vi "Script Add Custom Error.vi"(5 "Error Code":i32, 6 "Error Description":string, 7 "Error Name":string="TESTING.vi", 8 "error in":errorcluster, 9 "Error Arguments Window Ref":refnum<vi>, 10 "DQMH Lib Ref":refnum<vi>, 11 "Module type":T1) -> (0 "error out":errorcluster)   [LabVIEW 2019, in "Panther Dashboard.lvlib"]
uses:
  Panther Dashboard.lvlib
  Module type--enum.ctl
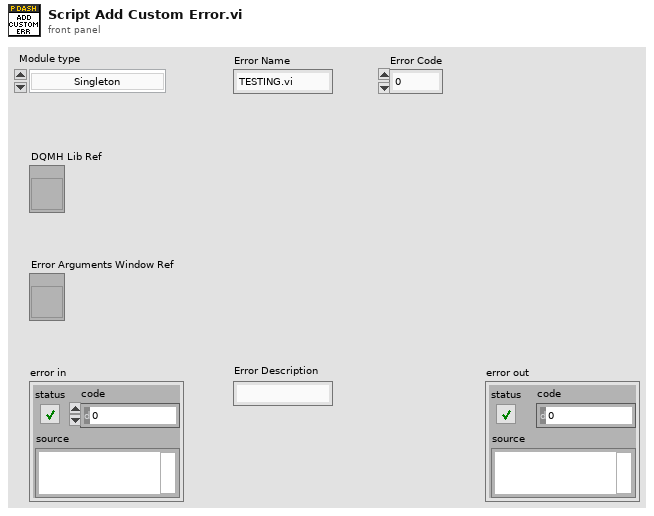
[diagram p1: front panel]
types:
  T1 = typedef "Panther Dashboard.lvlib/Module type--enum.ctl" = enum16{"Singleton", "Cloneable"}
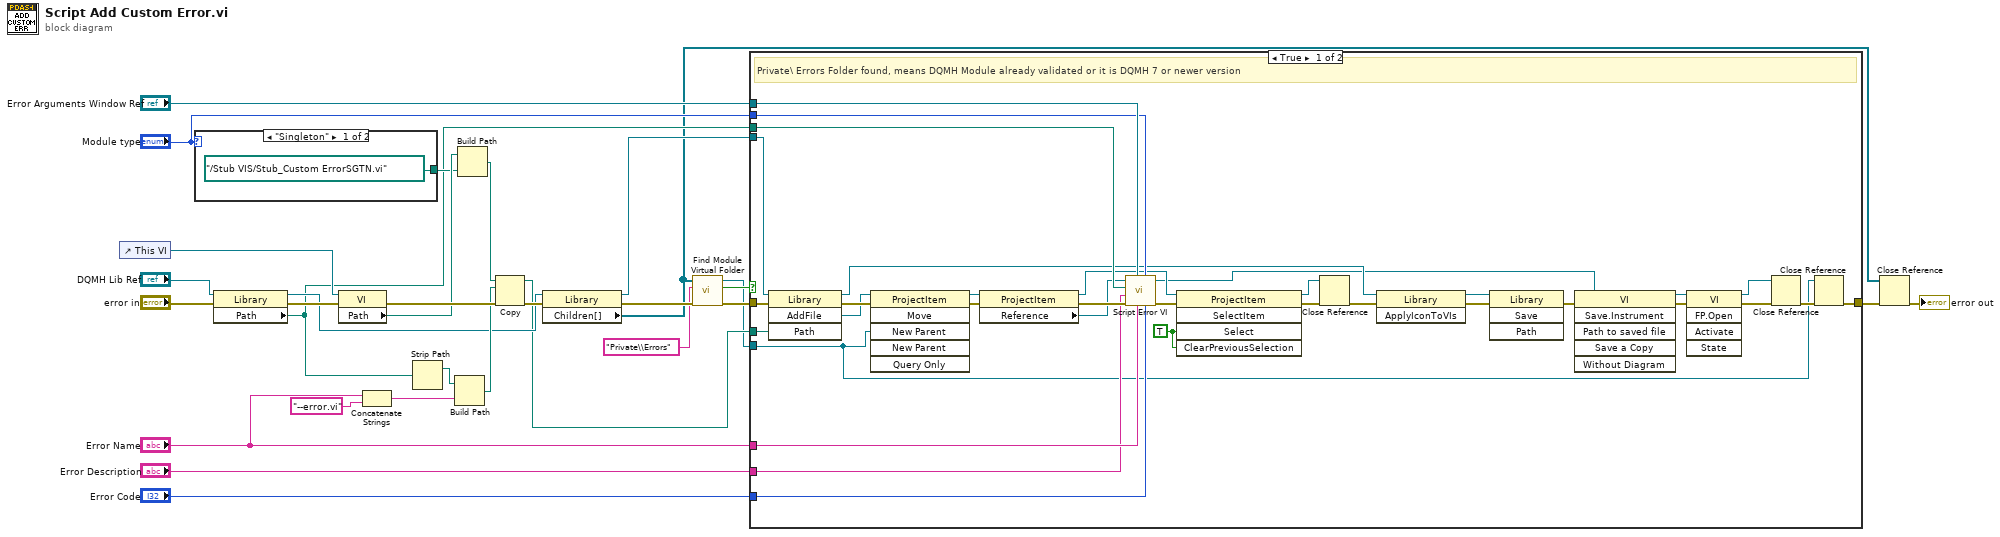
[diagram p0: block diagram]
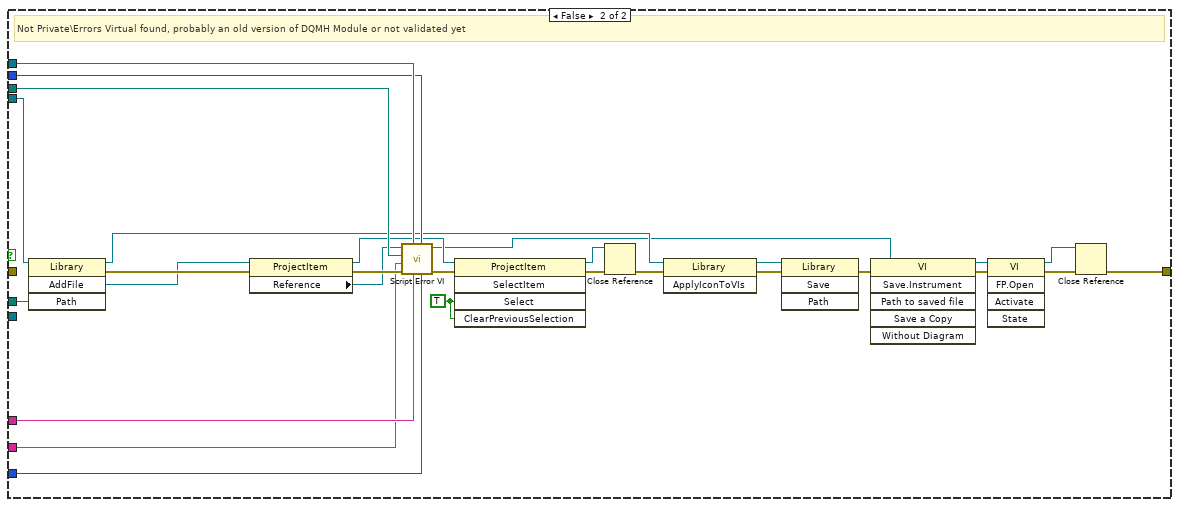
[diagram p2: hidden frame]
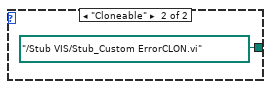
[diagram p3: hidden frame]
diagram:
  n1 = control-ref of="This VI"() -> (w20:refnum<vi>)
  n2 = case shown="\"Singleton\"" "Module type" {
    tunnel: [path "../Stub VIS/Stub_Custom ErrorSGTN.vi" path "../Stub VIS/Stub_Custom ErrorCLON.vi"] -> w18
    frame "Singleton" {
    }
    frame "Cloneable" {
    }
  }
  n3 = property class="Library"(reference="DQMH Lib Ref", error in="error in") -> (reference out=w13:refnum<vi>, error out=w28:errorcluster, "Path"=w11:path)
  n4 = property class="VI"(reference=w20, error in=w28) -> (error out=w29:errorcluster, "Path"=w19:path)  [unwired: 1 out]
  n5 = Concatenate Strings("Error Name", "--error.vi" ("input 1")) -> (w22:string)
  n6 = Strip Path(path=w11) -> (stripped path=w14:path)  [unwired: 1 out]
  n7 = Build Path(base path=w14, name or relative path=w22) -> (appended path=w21:path)
  n8 = Build Path(base path=w19, name or relative path=w18) -> (appended path=w17:path)
  n9 = Copy(8:w29, 10:w21, 11:w17) -> (0:w27:errorcluster, 3:w12:path)  [unwired: 2 in, 1 out]
  n10 = property class="Library"(reference=w13, error in=w27) -> (reference out=w16:refnum<vi>, error out=w24:errorcluster, "Children[]"=w4:refnum<vi>[])
  n11 = call "Find Module Virtual Folder.vi"("error in"=w24, "Virtual Folder"="Private\\Errors", "Children[]"=w4) -> ("error out"=w23:errorcluster, "Found?"=w3:bool, "ProjectItem out"=w2:refnum<vi>)  [unwired: 6 in]
  n12 = case shown="True" w3 {
    tunnel: [w63 w85] -> w30
    tunnel: w16 -> [w51 w82]
    tunnel: w12 -> [w52 w83]
    tunnel: w11 -> [w48 w80]
    tunnel: "Error Name" -> [w40 w72]
    tunnel: "Error Code" -> [w47 w79]
    tunnel: "Error Arguments Window Ref" -> [w45 w77]
    tunnel: "Module type" -> [w44 w76]
    tunnel: "Error Description" -> [w34 w66]
    tunnel: w2 -> [w33 _]
    tunnel: w23 -> [w53 _]
    frame True {
      w41 = TRUE ("Select")
      # "Private\\ Errors Folder found, means DQMH Module already validated or it is DQMH 7 or newer version"
      n13 = invoke class="Library" method="AddFile"(reference=w51, error in=w53, "Path"=w52) -> (reference out=w39:refnum<vi>, error out=w64:errorcluster, "AddFile"=w50:refnum<vi>)  [unwired: 1 in, 1 out]
      n14 = invoke class="ProjectItem" method="Move"(reference=w50, error in=w64, "New Parent"=w33) -> (reference out=w49:refnum<vi>, error out=w65:errorcluster)  [unwired: 3 in, 4 out]
      n15 = property class="ProjectItem"(reference=w49, error in=w65) -> (reference out=w43:refnum<vi>, error out=w60:errorcluster, "Reference"=w46:refnum<vi>)
      n16 = call "Script Error VI.vi"("Error Code"=w47, "Module type"=w44, "Error Name"=w40, "Error Arguments Window Ref"=w45, "error in"=w60, "Error Description"=w34, "Library Path"=w48, "VI Ref Error in"=w46) -> ("error out"=w62:errorcluster, "Custom Error VI Ref"=w36:refnum<vi>)  [unwired: 2 in]
      n17 = invoke class="ProjectItem" method="SelectItem"(reference=w43, error in=w62, "Select"=w41, "ClearPreviousSelection"=w41) -> (reference out=w42:refnum<vi>, error out=w61:errorcluster)  [unwired: 1 in, 3 out]
      n18 = Close Reference(reference=w42, error in (no error)=w61) -> (error out=w59:errorcluster)
      n19 = invoke class="Library" method="ApplyIconToVIs"(reference=w39, error in=w59) -> (reference out=w38:refnum<vi>, error out=w58:errorcluster)  [unwired: 1 in, 1 out]
      n20 = invoke class="Library" method="Save"(reference=w38, error in=w58) -> (error out=w57:errorcluster)  [unwired: 2 in, 3 out]
      n21 = invoke class="VI" method="Save.Instrument"(reference=w36, error in=w57) -> (reference out=w35:refnum<vi>, error out=w54:errorcluster)  [unwired: 4 in, 4 out]
      n22 = invoke class="VI" method="FP.Open"(reference=w35, error in=w54) -> (reference out=w37:refnum<vi>, error out=w56:errorcluster)  [unwired: 3 in, 3 out]
      n23 = Close Reference(reference=w37, error in (no error)=w56) -> (error out=w55:errorcluster)
      n24 = Close Reference(reference=w33, error in (no error)=w55) -> (error out=w63:errorcluster)
    }
    frame False {
      w73 = TRUE ("Select")
      # "Not Private\\Errors Virtual found, probably an old version of DQMH Module or not validated yet"
      n25 = invoke class="Library" method="AddFile"(reference=w82, "Path"=w83) -> (reference out=w71:refnum<vi>, error out=w93:errorcluster, "AddFile"=w81:refnum<vi>)  [unwired: 2 in, 1 out]
      n26 = property class="ProjectItem"(reference=w81, error in=w93) -> (reference out=w75:refnum<vi>, error out=w90:errorcluster, "Reference"=w78:refnum<vi>)
      n27 = call "Script Error VI.vi"("Error Code"=w79, "Module type"=w76, "Error Name"=w72, "Error Arguments Window Ref"=w77, "error in"=w90, "Error Description"=w66, "Library Path"=w80, "VI Ref Error in"=w78) -> ("error out"=w92:errorcluster, "Custom Error VI Ref"=w68:refnum<vi>)  [unwired: 2 in]
      n28 = invoke class="ProjectItem" method="SelectItem"(reference=w75, error in=w92, "Select"=w73, "ClearPreviousSelection"=w73) -> (reference out=w74:refnum<vi>, error out=w91:errorcluster)  [unwired: 1 in, 3 out]
      n29 = Close Reference(reference=w74, error in (no error)=w91) -> (error out=w89:errorcluster)
      n30 = invoke class="Library" method="ApplyIconToVIs"(reference=w71, error in=w89) -> (reference out=w70:refnum<vi>, error out=w88:errorcluster)  [unwired: 1 in, 1 out]
      n31 = invoke class="Library" method="Save"(reference=w70, error in=w88) -> (error out=w87:errorcluster)  [unwired: 2 in, 3 out]
      n32 = invoke class="VI" method="Save.Instrument"(reference=w68, error in=w87) -> (reference out=w67:refnum<vi>, error out=w84:errorcluster)  [unwired: 4 in, 4 out]
      n33 = invoke class="VI" method="FP.Open"(reference=w67, error in=w84) -> (reference out=w69:refnum<vi>, error out=w86:errorcluster)  [unwired: 3 in, 3 out]
      n34 = Close Reference(reference=w69, error in (no error)=w86) -> (error out=w85:errorcluster)
    }
  }
  n35 = Close Reference(reference=w4, error in (no error)=w30) -> (error out=→"error out":errorcluster)
